vi "Execute.vi"(8 "Error In":errorcluster, 10 "Source":string, 11 "Function In":refnum<class "Function.lvclass">) -> (0 "Error Out":errorcluster, 2 "Nodes":refnum<class "Abstract.lvclass">[](array[class]), 3 "Function Out":refnum<class "Function.lvclass">)   [LabVIEW 2018, in "Toolkit.lvlib" / "Data.lvlib" / "Function.lvclass"]
uses:
  Function.lvclass
  Low-Level/Nodes/Abstract/Abstract.lvclass
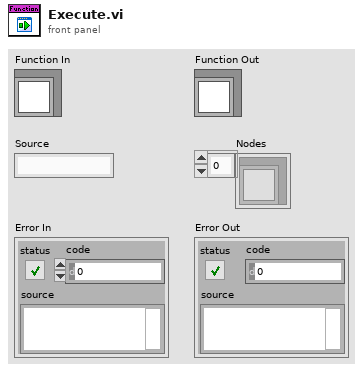
[diagram p1: front panel]
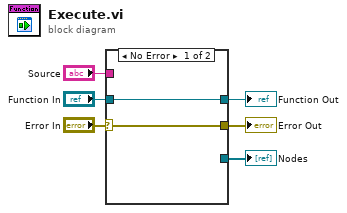
[diagram p0: block diagram]
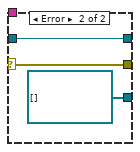
[diagram p2: hidden frame]
diagram:
  n1 = case shown="No Error" "Error In" {
    selector: "Error In" -> [w7 w10]
    tunnel: "Function In" -> [w8 w11]
    tunnel: [w8 w11] -> w4
    tunnel: [w7 w10] -> w3
    tunnel: "Source" -> [_ _]
    tunnel: [_ refnum<class "Abstract.lvclass">[] [] ("Nodes")] -> w1
    frame No Error {
    }
    frame Error {
    }
  }
  "Function Out" <- w4
  "Error Out" <- w3
  "Nodes" <- w1
